vi "SwissSPAD Live_Internal Data Storage.vi"(6 "Get(F)/Set":bool, 7 "SS2 Live Data":T3, 8 "Error In":errorcluster, 11 "Variant":variant) -> (0 "Error Out":errorcluster, 1 "Found/Replaced?":bool, 3 "Variant":variant)   [LabVIEW 2021]
uses:
  SwissSPAD Live_Internal Data List.ctl
  SwissSPAD Live_File Saving Task Information.ctl
  73672683-f5cc-4f44-afc7-723f83c649f1.vi
panel:
  in  "Histogram Window is Open":bool
  in  "Histogram Cursor Locations":cluster{"Min Cursor":dbl, "Max Cursor":dbl}
  in  "# FPGA Reset Attempts":i32
  in  "Current Image ROI Descriptor":T1 {"Contours"."Type" items=["No Selection", "Point", "Line", "Rectangle", "Oval", "Polygon", "Freehand Region", "Annulus", "Unused2", "Unused3", "Broken Line", "Freehand Line", "Rotated Rectangle"]}
  in  "File Saving Tasks Information":T2[](array[typedef])
  in  "Number of pending file saving tasks":i32
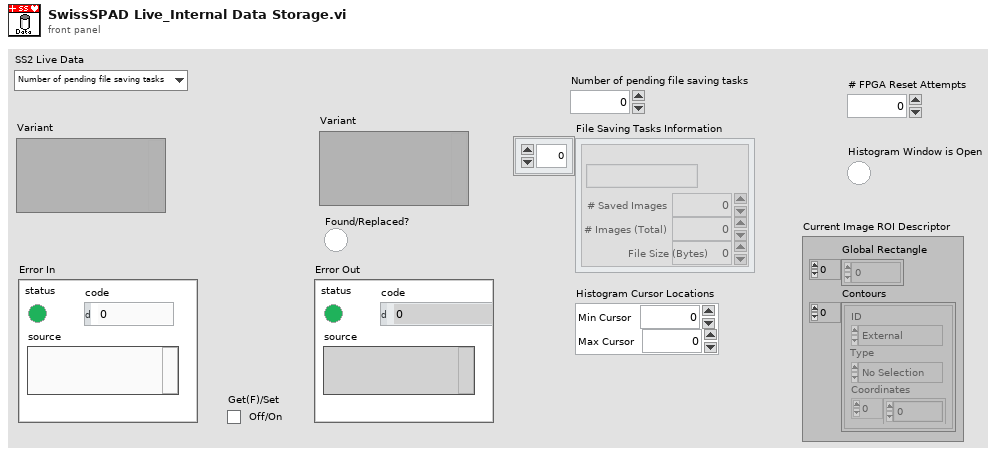
[diagram p1: front panel]
types:
  T1 = typedef "ROI Descriptor" = cluster{"Global Rectangle":i32[], "Contours":cluster{"ID":enum32{"External", "Internal"}, "Type":u32, "Coordinates":i32[]}[]}
  T2 = typedef "SwissSPAD Live_File Saving Task Information.ctl" = cluster{"File Path::n":string, "# Saved Images":i32, "# Images (Total)":i32, "File Size (Bytes)":i64}
  T3 = typedef "SwissSPAD Live_Internal Data List.ctl" = enum16{"Number of pending file saving tasks", "File Saving Tasks Information", "Current Image ROI Information", "# FPGA Reset Attempts", "Histogram Cursor Locations", "Histogram Window is Open"}
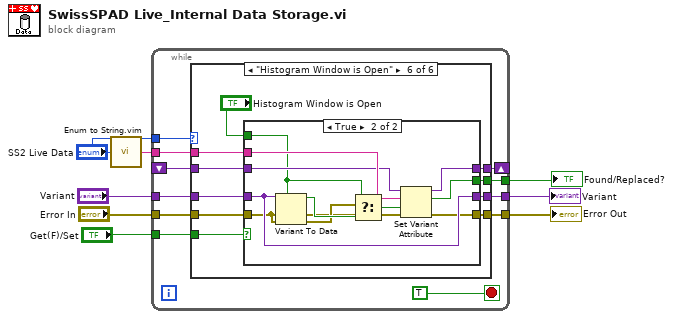
[diagram p0: block diagram]
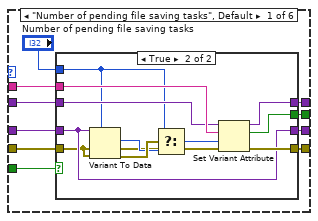
[diagram p2: hidden frame]
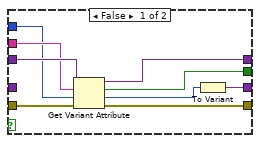
[diagram p3: hidden frame]
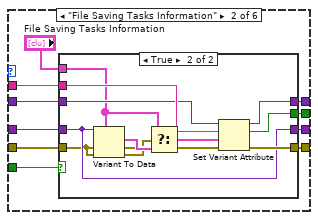
[diagram p4: hidden frame]
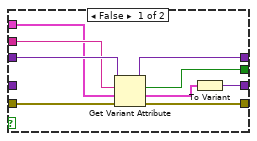
[diagram p5: hidden frame]
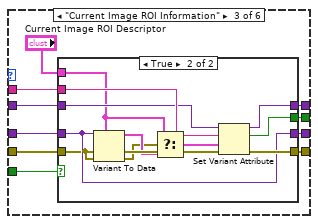
[diagram p6: hidden frame]
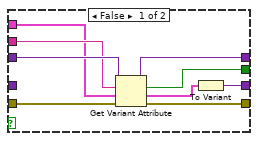
[diagram p7: hidden frame]
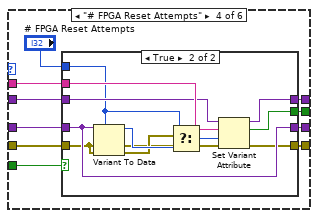
[diagram p8: hidden frame]
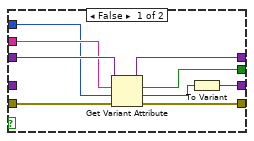
[diagram p9: hidden frame]
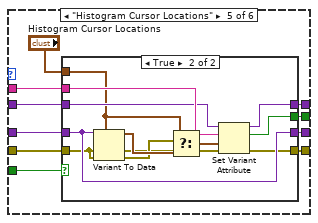
[diagram p10: hidden frame]
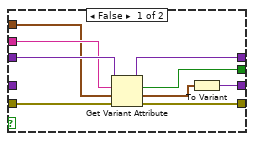
[diagram p11: hidden frame]
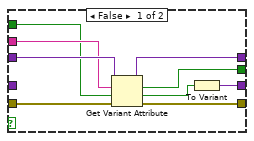
[diagram p12: hidden frame]
diagram:
  n1 = call "Enum to String.vim"("Enum"="SS2 Live Data") -> ("String"=w6:string)
  n2 = while {
    tunnel: "Get(F)/Set" -> [w18]
    shift-right: [w14] -> _
    shift-left: _ -> [w13]
    tunnel: "Variant" -> [w17]
    tunnel: w6 -> [w16]
    tunnel: "Error In" -> [w15]
    tunnel: [w12] -> w4
    tunnel: [w11] -> w3
    tunnel: [w10] -> w2
    tunnel: "SS2 Live Data" -> [w9]
    stop <- TRUE stop-if-true
    n3 = case shown="\"Histogram Window is Open\"" w9 {
      tunnel: w18 -> [w29 w59 w89 w119 w148 w177]
      tunnel: w17 -> [w28 w58 w88 w118 w147 w176]
      tunnel: w16 -> [w27 w57 w87 w117 w146 w175]
      tunnel: w15 -> [w26 w56 w86 w116 w145 w174]
      tunnel: [w25 w55 w85 w115 w144 w173] -> w14
      tunnel: w13 -> [w24 w54 w84 w114 w143 w172]
      tunnel: [w23 w53 w83 w113 w142 w171] -> w12
      tunnel: [w22 w52 w82 w112 w141 w170] -> w11
      tunnel: [w21 w51 w81 w111 w140 w169] -> w10
      frame "Number of pending file saving tasks", Default {
        n4 = case shown="True" w29 {
          tunnel: w28 -> [_ w44]
          tunnel: w27 -> [w36 w49]
          tunnel: w26 -> [w35 w39]
          tunnel: [w37 w48] -> w25
          tunnel: w24 -> [w38 w47]
          tunnel: [w34 w46] -> w23
          tunnel: [w31 w44] -> w22
          tunnel: [w32 w45] -> w21
          tunnel: "Number of pending file saving tasks" -> [w30 w41]
          frame False {
            n5 = Get Variant Attribute(Variant=w38, name=w36, default value (empty Variant)=w30, error in=w35) -> (duplicate Variant=w37:variant, found=w32:bool, value=w33:i32, error out=w34:errorcluster)
            n6 = To Variant(anything=w33) -> (Variant=w31:variant)
          }
          frame True {
            n7 = Variant To Data(error in=w39, type=w41, Variant=w44) -> (data=w42:i32, error out=w43:errorcluster)
            n8 = Select(t=w41, s=w43, f=w42) -> (s? t:f=w40:i32)
            n9 = Set Variant Attribute(Variant=w47, name=w49, value=w40, error in=w39) -> (Variant out=w48:variant, replaced=w45:bool, error out=w46:errorcluster)
          }
        }
      }
      frame "File Saving Tasks Information" {
        n10 = case shown="True" w59 {
          tunnel: w58 -> [_ w74]
          tunnel: w57 -> [w66 w79]
          tunnel: w56 -> [w65 w71]
          tunnel: [w67 w78] -> w55
          tunnel: w54 -> [w68 w77]
          tunnel: [w64 w76] -> w53
          tunnel: [w61 w74] -> w52
          tunnel: [w62 w75] -> w51
          tunnel: "File Saving Tasks Information" -> [w60 w69]
          frame False {
            n11 = Get Variant Attribute(Variant=w68, name=w66, default value (empty Variant)=w60, error in=w65) -> (duplicate Variant=w67:variant, found=w62:bool, value=w63:T2[], error out=w64:errorcluster)
            n12 = To Variant(anything=w63) -> (Variant=w61:variant)
          }
          frame True {
            n13 = Variant To Data(error in=w71, type=w69, Variant=w74) -> (data=w73:T2[], error out=w70:errorcluster)
            n14 = Select(t=w69, s=w70, f=w73) -> (s? t:f=w72:T2[])
            n15 = Set Variant Attribute(Variant=w77, name=w79, value=w72, error in=w71) -> (Variant out=w78:variant, replaced=w75:bool, error out=w76:errorcluster)
          }
        }
      }
      frame "Current Image ROI Information" {
        n16 = case shown="True" w89 {
          tunnel: w88 -> [_ w104]
          tunnel: w87 -> [w96 w109]
          tunnel: w86 -> [w95 w102]
          tunnel: [w97 w108] -> w85
          tunnel: w84 -> [w98 w107]
          tunnel: [w94 w106] -> w83
          tunnel: [w91 w104] -> w82
          tunnel: [w92 w105] -> w81
          tunnel: "Current Image ROI Descriptor" -> [w90 w99]
          frame False {
            n17 = Get Variant Attribute(Variant=w98, name=w96, default value (empty Variant)=w90, error in=w95) -> (duplicate Variant=w97:variant, found=w92:bool, value=w93:T1, error out=w94:errorcluster)
            n18 = To Variant(anything=w93) -> (Variant=w91:variant)
          }
          frame True {
            n19 = Variant To Data(error in=w102, type=w99, Variant=w104) -> (data=w101:T1, error out=w100:errorcluster)
            n20 = Select(t=w99, s=w100, f=w101) -> (s? t:f=w103:T1)
            n21 = Set Variant Attribute(Variant=w107, name=w109, value=w103, error in=w102) -> (Variant out=w108:variant, replaced=w105:bool, error out=w106:errorcluster)
          }
        }
      }
      frame "# FPGA Reset Attempts" {
        n22 = case shown="True" w119 {
          tunnel: w118 -> [_ w134]
          tunnel: w117 -> [w126 w138]
          tunnel: w116 -> [w125 w129]
          tunnel: [w127 w137] -> w115
          tunnel: w114 -> [w128 w136]
          tunnel: [w124 w129] -> w113
          tunnel: [w121 w134] -> w112
          tunnel: [w122 w135] -> w111
          tunnel: "# FPGA Reset Attempts" -> [w120 w131]
          frame False {
            n23 = Get Variant Attribute(Variant=w128, name=w126, default value (empty Variant)=w120, error in=w125) -> (duplicate Variant=w127:variant, found=w122:bool, value=w123:i32, error out=w124:errorcluster)
            n24 = To Variant(anything=w123) -> (Variant=w121:variant)
          }
          frame True {
            n25 = Variant To Data(error in=w129, type=w131, Variant=w134) -> (data=w133:i32, error out=w130:errorcluster)
            n26 = Select(t=w131, s=w130, f=w133) -> (s? t:f=w132:i32)
            n27 = Set Variant Attribute(Variant=w136, name=w138, value=w132) -> (Variant out=w137:variant, replaced=w135:bool)  [unwired: 1 in, 1 out]
          }
        }
      }
      frame "Histogram Cursor Locations" {
        n28 = case shown="True" w148 {
          tunnel: w147 -> [_ w163]
          tunnel: w146 -> [w155 w167]
          tunnel: w145 -> [w154 w158]
          tunnel: [w156 w166] -> w144
          tunnel: w143 -> [w157 w165]
          tunnel: [w153 w158] -> w142
          tunnel: [w150 w163] -> w141
          tunnel: [w151 w164] -> w140
          tunnel: "Histogram Cursor Locations" -> [w149 w160]
          frame False {
            n29 = Get Variant Attribute(Variant=w157, name=w155, default value (empty Variant)=w149, error in=w154) -> (duplicate Variant=w156:variant, found=w151:bool, value=w152:cluster{"Min Cursor":dbl, "Max Cursor":dbl}, error out=w153:errorcluster)
            n30 = To Variant(anything=w152) -> (Variant=w150:variant)
          }
          frame True {
            n31 = Variant To Data(error in=w158, type=w160, Variant=w163) -> (data=w162:cluster{"Min Cursor":dbl, "Max Cursor":dbl}, error out=w159:errorcluster)
            n32 = Select(t=w160, s=w159, f=w162) -> (s? t:f=w161:cluster{"Min Cursor":dbl, "Max Cursor":dbl})
            n33 = Set Variant Attribute(Variant=w165, name=w167, value=w161) -> (Variant out=w166:variant, replaced=w164:bool)  [unwired: 1 in, 1 out]
          }
        }
      }
      frame "Histogram Window is Open" {
        n34 = case shown="True" w177 {
          tunnel: w176 -> [_ w192]
          tunnel: w175 -> [w184 w196]
          tunnel: w174 -> [w183 w187]
          tunnel: [w185 w195] -> w173
          tunnel: w172 -> [w186 w194]
          tunnel: [w182 w187] -> w171
          tunnel: [w179 w192] -> w170
          tunnel: [w180 w193] -> w169
          tunnel: "Histogram Window is Open" -> [w178 w189]
          frame False {
            n35 = Get Variant Attribute(Variant=w186, name=w184, default value (empty Variant)=w178, error in=w183) -> (duplicate Variant=w185:variant, found=w180:bool, value=w181:bool, error out=w182:errorcluster)
            n36 = To Variant(anything=w181) -> (Variant=w179:variant)
          }
          frame True {
            n37 = Variant To Data(error in=w187, type=w189, Variant=w192) -> (data=w191:bool, error out=w188:errorcluster)
            n38 = Select(t=w189, s=w188, f=w191) -> (s? t:f=w190:bool)
            n39 = Set Variant Attribute(Variant=w194, name=w196, value=w190) -> (Variant out=w195:variant, replaced=w193:bool)  [unwired: 1 in, 1 out]
          }
        }
      }
    }
  }
  "Error Out" <- w4
  "Variant" <- w3
  "Found/Replaced?" <- w2
